vi "Write Scheduled.vi"(4 "size (unlimited)":i32, 7 "scheduled time":timestamp, 9 "last element? (F)":bool, 10 "element":T1, 11 "element valid? (T)":bool=TRUE) -> (2 "channel":T2, 3 "count":i32, 5 "actual time":timestamp)   [LabVIEW 2017, in "Stream-t'WPI_EncoderType.ctl'.lvlib"]
doc: "Writes an element to a Stream channel at a scheduled time. The endpoint waits until the scheduled time and continues waiting if the channel is full at the scheduled time."
uses:
  <extravilib>/ChannelInstances/Stream-t'WPI_EncoderType.ctl'.lvlib
  <extravilib>/ChannelInstances/Stream-t'WPI_EncoderType.ctl'/)Channel.ctl
  <vilib>/Rock Robotics/WPI/Encoder/WPI_EncoderType.ctl
  <extravilib>/ChannelInstances/Stream-t'WPI_EncoderType.ctl'/Write With Abort.vi
  <extravilib>/ChannelInstances/Stream-t'WPI_EncoderType.ctl'/Endpoint.vi
  <resource>/ChannelSupport/_ChannelSupport/WaitIfNeeded.vi
  <extravilib>/ChannelInstances/Stream-t'WPI_EncoderType.ctl'/)Channel.vi
  <resource>/ChannelSupport/_ChannelSupport/_ChannelSupport.lvlib
  <resource>/ChannelSupport/_ChannelSupport/GetErrors/FpgaChannelWireNotSupported.xnode
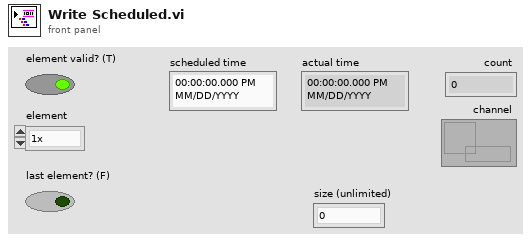
[diagram p1: front panel]
types:
  T1 = typedef "WPI_EncoderType.ctl" = enum16{"1x", "2x", "4x"}
  T2 = typedef "Stream-t'WPI_EncoderType.ctl'.lvlib/)Channel.ctl" = refnum<queue>
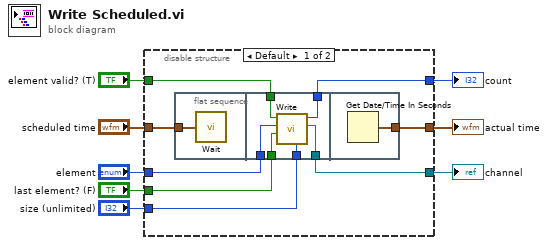
[diagram p0: block diagram]
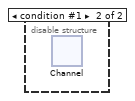
[diagram p2: hidden frame]
diagram:
  n1 = disable-structure shown="Default" {
    disable-tunnel: "scheduled time" -> [w16 _]
    disable-tunnel: [w15 _] -> w7
    disable-tunnel: "element" -> [w14 _]
    disable-tunnel: [w13 _] -> w5
    disable-tunnel: "size (unlimited)" -> [w12 _]
    disable-tunnel: "element valid? (T)" -> [w11 _]
    disable-tunnel: "last element? (F)" -> [w10 _]
    disable-tunnel: [w9 _] -> w1
    frame condition #0 (active) {
      n2 = flat-sequence {
        tunnel: w16 -> [w17]
        tunnel: w14 -> [w22]
        tunnel: [w21] -> w13
        tunnel: w12 -> [w23]
        tunnel: w11 -> [w20]
        tunnel: w10 -> [w19]
        tunnel: [w18] -> w9
        tunnel: [w24] -> w15
        frame #0 {
          n3 = call <resource>:"Wait.vi"("desired time"=w17) -> ()  [unwired: 2 out]
        }
        frame #1 {
          n4 = call <extravilib>:"Write.vi"("size (unlimited)"=w23, "last element? (F)"=w19, "element"=w22, "element valid? (T)"=w20) -> ("channel"=w21:T2, "count"=w18:i32)  [unwired: 5 in, 1 out]
        }
        frame #2 {
          n5 = Get Date/Time In Seconds() -> (seconds since 1Jan1904=w24:timestamp)
        }
      }
    }
    frame condition #1 {
      n6 = xnode "Channel"() -> ()
    }
  }
  "channel" <- w5
  "actual time" <- w7
  "count" <- w1
